vi "Integer NOT Gate (SubVI).vi"(1 "Input State(Integer)":dbl) -> (0 "Output State (Integer)":dbl)   [LabVIEW 2015]
panel:
  # "Output = Not Input"
  # "If \"Input State (Integer)\" = 1 Then \"Output State (Integer)\" = 0"
  # "If \"Input State (Integer)\" = 0 Then \"Output State (Integer)\" = 1"
  # "Basically Its a \"Not Gate\" Which Accepts Integer(0,1) As Input & Gives Output In Integer(0,1) [[ It is not boolean NOT gate ]]"
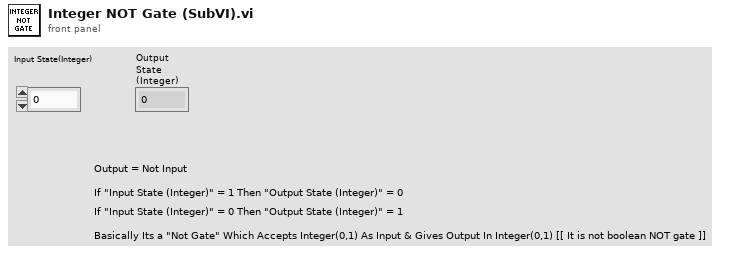
[diagram p1: front panel]
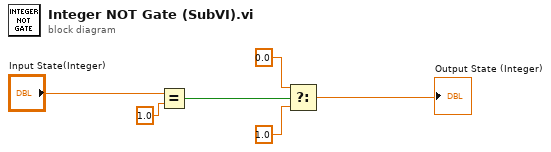
[diagram p0: block diagram]
diagram:
  n1 = Equal?(x="Input State(Integer)", y=1.0) -> (x = y?=w3:bool)
  n2 = Select(t=0.0, s=w3, f=1.0) -> (s? t:f=→"Output State (Integer)":dbl)
